vi "ASI_serialWhere_ALL_AXIS.vi"(4 "error in (no error)":errorcluster, 7 "VISA resource name":refnum<visa-resource-name>="COM7") -> (0 "error out":errorcluster, 1 "Z":dbl format="%.2f", 2 "Y":dbl format="%.2f", 3 "X":dbl format="%#.1f")   [LabVIEW 2015]
doc: "Establishes connection with configured port (default = COM1).\nSends command MOVE X=x Y=y where x and y are integers denoting 10ths of a micron.\nSub-VI SerialWaitForStatusN.vi polls controller with STATUS command until 'N' (not busy) status is returned, or until a configured maximum number of unsuccessful tries (default = 400).\nDisconnects from configured port."
uses:
  <vilib>/Instr/_visa.llb/VISA Flush IO Buffer Mask.ctl
panel:
  out "read buffer":string
  # "Note: This VI ships with 100 ms as the default timeout value. That means that the\nVI will listen to the MS2000 for up to 100 ms after sending a command.\nMS2000 terminates its reply with CR. This VI is configured by VISA Configure Serial Port.vi\nto stop listening when it receives a CR (decimal 13). \nNormally the MS2000 completes its reply within the 100 ms timeout. This timeout value\ncan be adjusted down for faster performance.\nHowever, if too low, then the VI may not wait long enough for the MS2000\nto reply to the command."
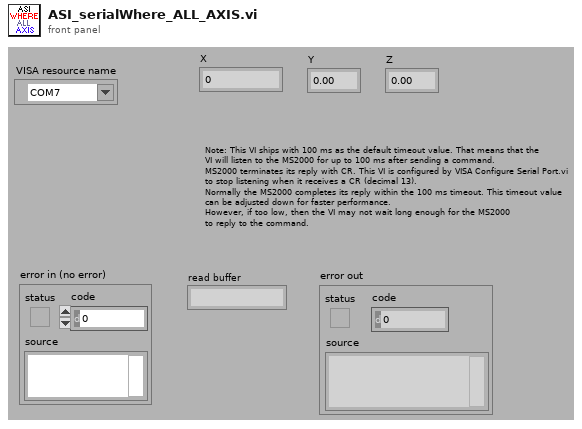
[diagram p1: front panel]
types:
  T1 = typedef "VISA Flush IO Buffer Mask.ctl" = u16
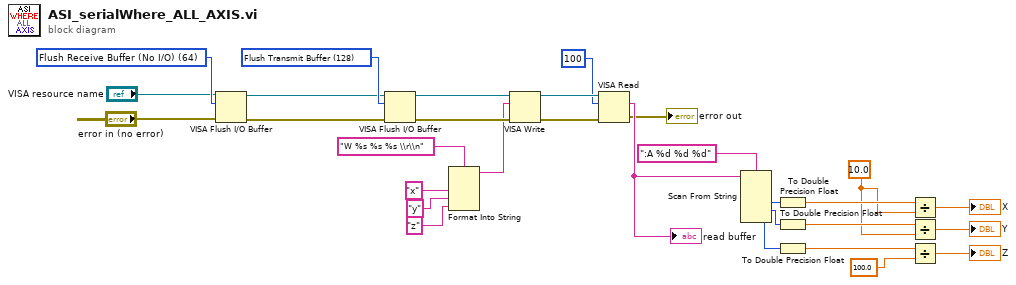
[diagram p0: block diagram]
diagram:
  w1 = 10.0
  w21 = T1 64 items=["Flush Receive Buffer"=16, "Write Transmit Buffer to Device"=32, "Flush Receive Buffer (No I/O)"=64, "Flush Transmit Buffer"=128] ("Mask")
  w22 = T1 128 items=["Flush Receive Buffer"=16, "Write Transmit Buffer to Device"=32, "Flush Receive Buffer (No I/O)"=64, "Flush Transmit Buffer"=128] ("Mask")
  n1 = VISA Flush I/O Buffer(VISA resource name="VISA resource name", mask (16)=w21, error in (no error)="error in (no error)") -> (VISA resource name out=w18:refnum<visa-resource-name>, error out=w23:errorcluster)
  n2 = VISA Flush I/O Buffer(VISA resource name=w18, mask (16)=w22, error in (no error)=w23) -> (VISA resource name out=w20:refnum<visa-resource-name>, error out=w19:errorcluster)
  n3 = Format Into String "Format Into String"(format string="W %s %s %s \\r\\n", "x" ("input 1"), "y" ("input 2"), "z" ("input 3")) -> (resulting string=w15:string)  [unwired: 2 in, 1 out]
  n4 = VISA Write(VISA resource name=w20, write buffer=w15, error in (no error)=w19) -> (VISA resource name out=w30:refnum<visa-resource-name>, error out=w29:errorcluster)  [unwired: 1 out]
  n5 = VISA Read(VISA resource name=w30, byte count=u32 100, error in (no error)=w29) -> (read buffer=w27:string, error out=→"error out":errorcluster)  [unwired: 2 out]
  "read buffer" <- w27
  n6 = Scan From String "Scan From String"(format string=":A %d %d %d", input string=w27) -> (output 1=w9:i32, output 2=w11:i32, output 3=w10:i32)  [unwired: 5 in, 3 out]
  n7 = To Double Precision Float(number=w9) -> (double precision float=w2:dbl)
  n8 = To Double Precision Float(number=w11) -> (double precision float=w3:dbl)
  n9 = To Double Precision Float(number=w10) -> (double precision float=w4:dbl)
  n10 = Divide(x=w2, y=w1) -> (x/y=→"X":dbl)
  n11 = Divide(x=w3, y=w1) -> (x/y=→"Y":dbl)
  n12 = Divide(x=w4, y=100.0) -> (x/y=→"Z":dbl)
